vi "recondense_Check_Queue.vi"(7 "error in (no error)":errorcluster, 10 "Queue":refnum<queue> caption="5T Queue") -> (0 "error out":errorcluster, 1 "Recondense-Control":T1, 3 "New Entries?":bool)   [LabVIEW 2019]
uses:
  Brosowski/Borowski-Control-Cluster.ctl
panel:
  out "Numeric":i32
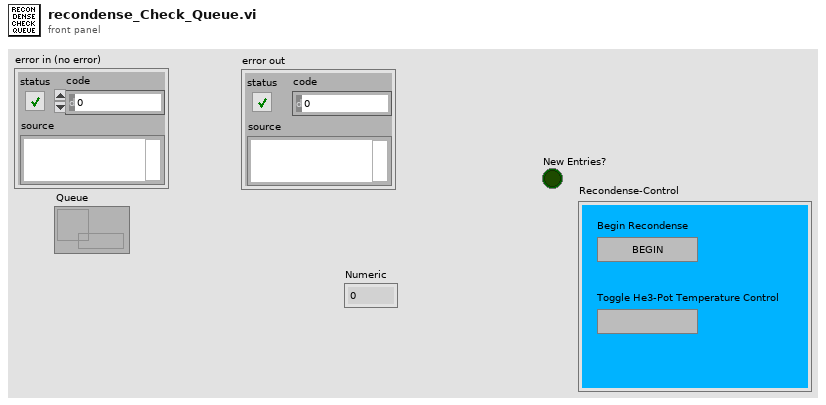
[diagram p1: front panel]
types:
  T1 = typedef "Borowski-Control-Cluster.ctl" = cluster{"Begin Recondense":bool, "Toggle He3-Pot Temperature Control":bool}
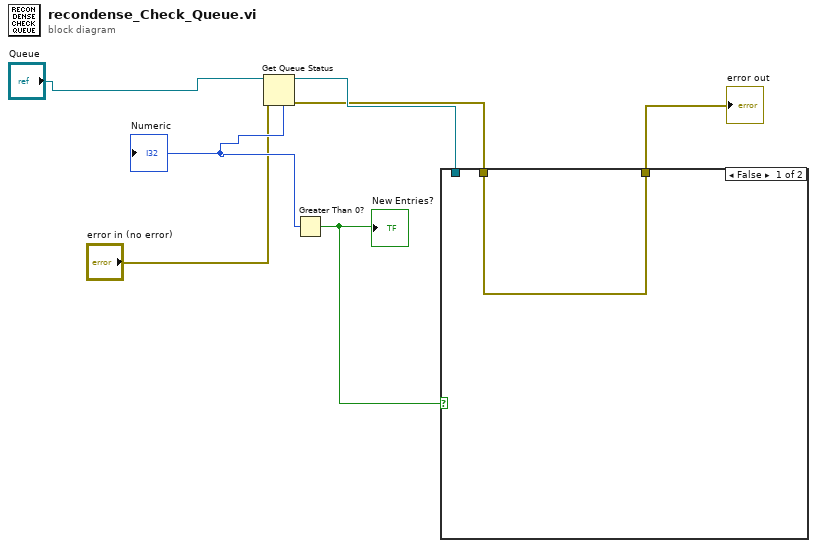
[diagram p0: block diagram]
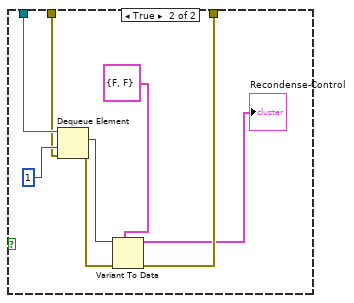
[diagram p2: hidden frame]
diagram:
  n1 = Get Queue Status(queue="Queue", error in (no error)="error in (no error)") -> (queue out=w6:refnum<queue>, error out=w4:errorcluster, # elements in queue=w7:i32)  [unwired: 1 in, 5 out]
  "Numeric" <- w7
  n2 = Greater Than 0?(x=w7) -> (x > 0?=w5:bool)
  "New Entries?" <- w5
  n3 = case shown="False" w5 {
    tunnel: w6 -> [_ w14]
    tunnel: w4 -> [w8 w13]
    tunnel: [w8 w11] -> w2
    frame False {
    }
    frame True {
      n4 = Dequeue Element(queue=w14, timeout in ms (-1)=1, error in (no error)=w13) -> (element=w15:variant, error out=w12:errorcluster)  [unwired: 2 out]
      n5 = Variant To Data(error in=w12, type=T1 {"Begin Recondense"=FALSE, "Toggle He3-Pot Temperature Control"=FALSE} ("Recondense-Control"), Variant=w15) -> (data=→"Recondense-Control":T1, error out=w11:errorcluster)
    }
  }
  "error out" <- w2
